vi "test - Remove Filter - 1.vi"(8 "error in (no error)":errorcluster, 11 "TestCase in":refnum<class "Remove Filter Unit Test.lvclass">) -> (0 "error out":errorcluster, 3 "TestCase out":refnum<class "Remove Filter Unit Test.lvclass">)   [LabVIEW 2016, in "Assert API Components.lvlib" / "Assert Display.lvlib" / "Main Display.lvlib" / "Remove Filter Unit Test.lvclass"]
uses:
  Remove Filter Unit Test.lvclass
  Remove Filter Unit Test.lvclass/Remove Filter Unit Test.ctl
  <vilib>/addons/_JKI Toolkits/VI Tester/TestCase.llb/TestCase.lvclass
  Core/Main Display/Main Display/Main Display.lvclass
  Core/Main Display/Main Display.lvlib
  C:/Program Files (x86)/National Instruments/LabVIEW 2016/vi.lib/addons/_JKI Toolkits/VI Tester/TestCase.llb/TestCase.lvclass
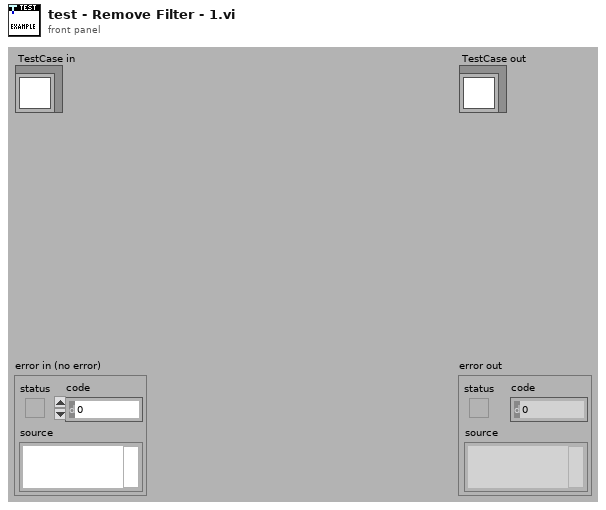
[diagram p1: front panel]
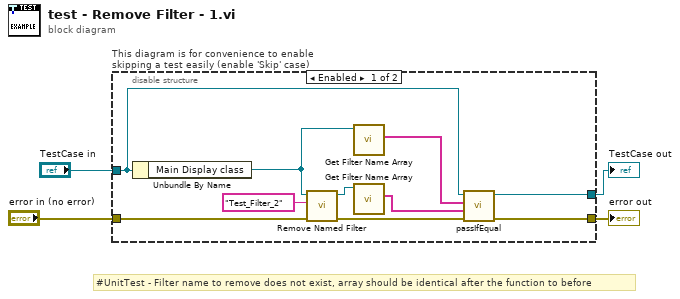
[diagram p0: block diagram]
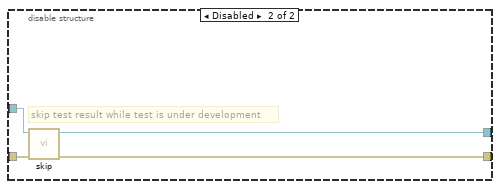
[diagram p2: hidden frame]
diagram:
  # "#UnitTest - Filter name to remove does not exist, array should be identical after the function to before"
  n1 = disable-structure "This diagram is for convenience to enable skipping a test easily (enable 'Skip' case)" shown="Enabled" {
    disable-tunnel: "TestCase in" -> [w12 w18]
    disable-tunnel: [w14 w16] -> w1
    disable-tunnel: [w13 w17] -> w3
    disable-tunnel: "error in (no error)" -> [w9 w15]
    frame Enabled {
      n2 = Unbundle By Name(w12) -> ("Main Display class"=w6:refnum<class "Main Display.lvclass">)
      n3 = call "Remove Named Filter.vi"("error in (no error)"=w9, "Filter Name"="Test_Filter_2", "Main Display in"=w6) -> ("error out"=w8:errorcluster, "Main Display out"=w10:refnum<class "Main Display.lvclass">)  [unwired: 7 in]
      n4 = call "Get Filter Name Array.vi"("Main Display in"=w6) -> ("Filter Name Array"=w5:string[])  [unwired: 10 in]
      n5 = call "Get Filter Name Array.vi"("Main Display in"=w10) -> ("Filter Name Array"=w7:string[])  [unwired: 10 in]
      n6 = call-dynamic "passIfEqual.vi"("error in (no error)"=w8, "y"=w7, "x"=w5, "TestCase in"=w12) -> ("error out"=w13:errorcluster, "TestCase out"=w14:refnum<class "Remove Filter Unit Test.lvclass">)  [unwired: 6 in]
    }
    frame Disabled {
      # "skip test result while test is under development"
      n7 = call <vilib>:"skip.vi"("error in (no error)"=w15, "TestCase in"=w18) -> ("error out"=w17:errorcluster, "TestCase out"=w16:refnum<class "Remove Filter Unit Test.lvclass">)  [unwired: 8 in]
    }
  }
  "error out" <- w3
  "TestCase out" <- w1
